vi "DB Tools List Tables.vi"(4 "error in (no error)":errorcluster, 7 "connection reference":T1) -> (0 "error out":errorcluster, 2 "tables":string[](array[string]), 3 "connection reference out":T1)   [LabVIEW 2017, in "NI_Database_API.lvlib"]
doc: "Lists the tables in the database identified by <B>connection reference</B>."
uses:
  <vilib>/addons/database/NI_Database_API.lvlib
  <vilib>/addons/database/Connection.llb/Conn ObjectReference.ctl
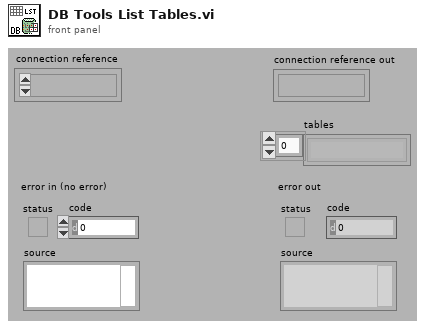
[diagram p1: front panel]
types:
  T1 = typedef "NI_Database_API.lvlib/Conn ObjectReference.ctl" = refnum<k1>
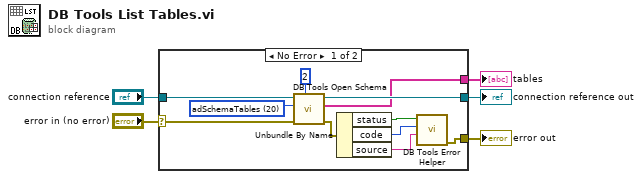
[diagram p0: block diagram]
diagram:
  n1 = case shown="No Error" "error in (no error)" {
    selector: "error in (no error)" -> [w6 w18]
    tunnel: "connection reference" -> [w16 w17]
    tunnel: [w15 w17] -> w4
    tunnel: [w12 _] -> w3
    tunnel: [w8 w18] -> w2
    frame No Error {
      w14 = 20 items=["adSchemaProviderSpecific"=-1, "adSchemaAsserts"=0, "adSchemaCatalogs"=1, "adSchemaCharacterSets"=2, "adSchemaCollations"=3, "adSchemaColumns"=4, "adSchemaCheckConstraints"=5, "adSchemaConstraintColumnUsage"=6, "adSchemaConstraintTableUsage"=7, "adSchemaKeyColumnUsage"=8, "adSchemaReferentialContraints, adSchemaReferentialConstraints"=9, "adSchemaTableConstraints"=10, "adSchemaColumnsDomainUsage"=11, "adSchemaIndexes"=12, "adSchemaColumnPrivileges"=13, "adSchemaTablePrivileges"=14, "adSchemaUsagePrivileges"=15, "adSchemaProcedures"=16, "adSchemaSchemata"=17, "adSchemaSQLLanguages"=18, "adSchemaStatistics"=19, "adSchemaTables"=20, "adSchemaTranslations"=21, "adSchemaProviderTypes"=22, "adSchemaViews"=23, "adSchemaViewColumnUsage"=24, "adSchemaViewTableUsage"=25, "adSchemaProcedureParameters"=26, "adSchemaForeignKeys"=27, "adSchemaPrimaryKeys"=28, "adSchemaProcedureColumns"=29, "adSchemaDBInfoKeywords"=30, "adSchemaDBInfoLiterals"=31, "adSchemaCubes"=32, "adSchemaDimensions"=33, "adSchemaHierarchies"=34, "adSchemaLevels"=35, "adSchemaMeasures"=36, "adSchemaProperties"=37, "adSchemaMembers"=38, "adSchemaTrustees"=39] ("schema")
      n2 = call <vilib>:"DB Tools Open Schema.vi"("column"=2, "error in (no error)"=w6, "Schema"=w14, "connection reference"=w16) -> ("error out"=w9:errorcluster, "schema data"=w12:string[], "connection reference out"=w15:T1)  [unwired: 1 in, 1 out]
      n3 = Unbundle By Name(w9) -> ("status"=w10:bool, "code"=w7:i32, "source"=w11:string)
      n4 = call <vilib>:"DB Tools Error Helper.vi"("source"=w11, "code"=w7, "status"=w10) -> ("error out"=w8:errorcluster)  [unwired: 1 in, 7 out]
    }
    frame Error {
    }
  }
  "connection reference out" <- w4
  "error out" <- w2
  "tables" <- w3
